vi "Event Create.vi"(9 "Event Actor":refnum<class "Event Actor.lvclass">, 10 "Alias":string, 11 "jettl Queue Actor in":refnum<class "jettl Queue Actor.lvclass">) -> (3 "jettl Queue Actor out":refnum<class "jettl Queue Actor.lvclass">)   [LabVIEW 2021, in "jettl.lvlib" / "jettl Queue Actor.lvclass"]
uses:
  jettl Queue Actor.lvclass
  Actor/Event Actor/Event Actor.lvclass
  Actor/Msg/Msg.lvclass
  jettl Queue Actor.lvclass/jettl Queue Actor.ctl
  jettl.lvlib
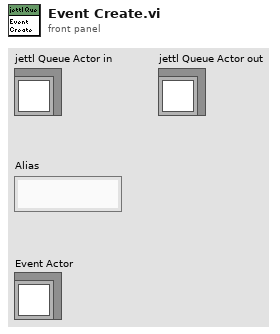
[diagram p1: front panel]
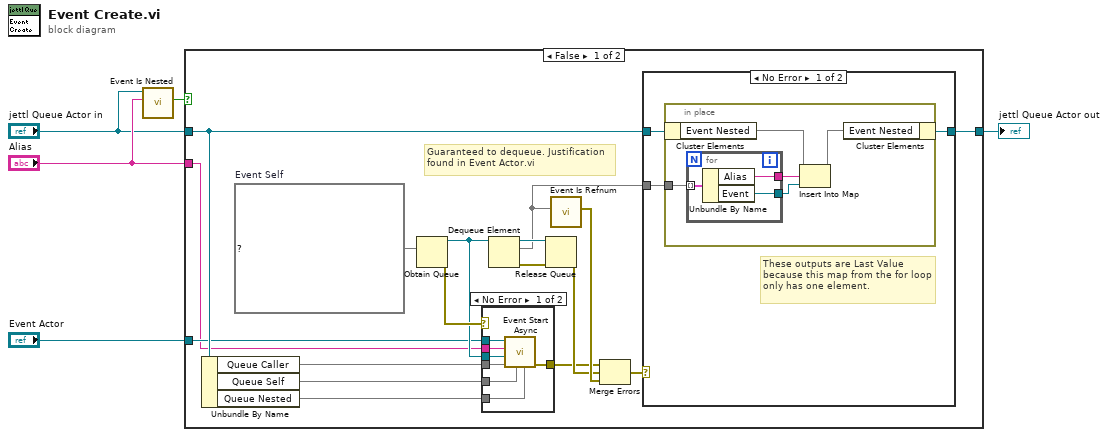
[diagram p0: block diagram]
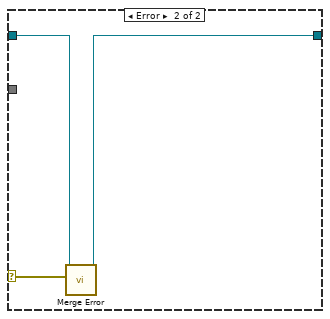
[diagram p3: hidden frame]
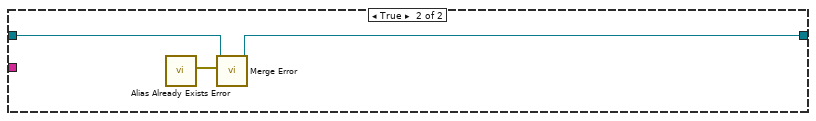
[diagram p4: hidden frame]
diagram:
  n1 = call-dynamic "Event Is Nested.vi"("Alias"="Alias", "jettl Queue Actor in"="jettl Queue Actor in") -> ("Event Is Nested?"=w3:bool)  [unwired: 9 in]
  n2 = case shown="False" w3 {
    tunnel: "Event Actor" -> [w15 _]
    tunnel: "jettl Queue Actor in" -> [w18 w47]
    tunnel: "Alias" -> [w14 _]
    tunnel: [w17 w46] -> w4
    frame False {
      w13 = map{string, refnum<data-value>} {}  # Event Self
      # "Guaranteed to dequeue. Justification found in Event Actor.vi"
      n3 = Unbundle By Name(w18) -> ("Queue Caller"=w8:map{string, refnum<data-value>}, "Queue Self"=w7:map{string, refnum<data-value>}, "Queue Nested"=w6:map{string, refnum<data-value>})
      n4 = Obtain Queue(element data type=w13) -> (queue out=w16:refnum<queue>, error out=w22:errorcluster)  [unwired: 4 in, 1 out]
      n5 = case shown="No Error" w22 {
        selector: w22 -> [_ w30]
        tunnel: [w23 w30] -> w9
        tunnel: w15 -> [w29 _]
        tunnel: w16 -> [w27 _]
        tunnel: w14 -> [w28 _]
        tunnel: w8 -> [w26 _]
        tunnel: w7 -> [w25 _]
        tunnel: w6 -> [w24 _]
        frame No Error {
          n6 = call "Event Start Async.vi"("Queue Nested"=w24, "Queue Self"=w25, "Queue Caller"=w26, "Queue of Event Self"=w27, "Event Self Alias"=w28, "Event Actor"=w29) -> ("error out"=w23:errorcluster)  [unwired: 5 in]
        }
        frame Error {
        }
      }
      n7 = Dequeue Element(queue=w16) -> (queue out=w20:refnum<queue>, element=w12:map{string, refnum<data-value>}, error out=w21:errorcluster)  [unwired: 2 in, 1 out]
      n8 = Release Queue(queue=w20, error in (no error)=w21) -> (error out=w10:errorcluster)  [unwired: 1 in, 2 out]
      n9 = call "Event Is Refnum.vi"("Event Self"=w12) -> ("Error"=w11:errorcluster)  [unwired: 10 in]
      n10 = Merge Errors(w9, w10, w11) -> (w19:errorcluster)
      n11 = case shown="No Error" w19 {
        selector: w19 -> [_ w42]
        tunnel: w18 -> [w33 w44]
        tunnel: [w32 w43] -> w17
        tunnel: w12 -> [w31 _]
        frame No Error {
          # "These outputs are Last Value because this map from the for loop only has one element."
          n12 = in-place {
            in-place-border: w31 -> [w36]
            n13 = in-place-cluster #1(w33) -> ("Event Nested"=w38:map{string, refnum<data-value>})
            n14 = for {
              tunnel: w36 -> [w41] mode=indexing
              tunnel: [w40] -> w35
              tunnel: [w39] -> w34
              n15 = Unbundle By Name(w41) -> ("Alias"=w40:string, "Event"=w39:refnum<data-value>)
            }
            n16 = Insert Into Map(map in=w38, key=w35, value=w34) -> (map out=w37:map{string, refnum<data-value>})  [unwired: 2 out]
            n17 = in-place-cluster #1("Event Nested"=w37) -> (w32:refnum<class "jettl Queue Actor.lvclass">)
          }
        }
        frame Error {
          n18 = call-dynamic "Merge Error.vi"("Error"=w42, "jettl Queue Actor in"=w44) -> ("jettl Queue Actor out"=w43:refnum<class "jettl Queue Actor.lvclass">)  [unwired: 9 in]
        }
      }
    }
    frame True {
      n19 = call "Alias Already Exists Error.vi"() -> ("Error"=w45:errorcluster)  [unwired: 11 in]
      n20 = call-dynamic "Merge Error.vi"("Error"=w45, "jettl Queue Actor in"=w47) -> ("jettl Queue Actor out"=w46:refnum<class "jettl Queue Actor.lvclass">)  [unwired: 9 in]
    }
  }
  "jettl Queue Actor out" <- w4
